vi "Start stream.vi"(10 "Channels to stream":string[](array[string]), 11 "Connection type":string) -> (0 "error out":errorcluster, 1 "ScansPerRead":i32, 2 "Actual ScanRate":dbl format="%.3f", 3 "Handle out":i32, 4 "Number of channels":i32)   [LabVIEW 2018]
panel:
  out "Stream channels":i32[](array[numeric])
  # "This sub VI opens a stream in Labjack. All the settings for the stream are also set here."
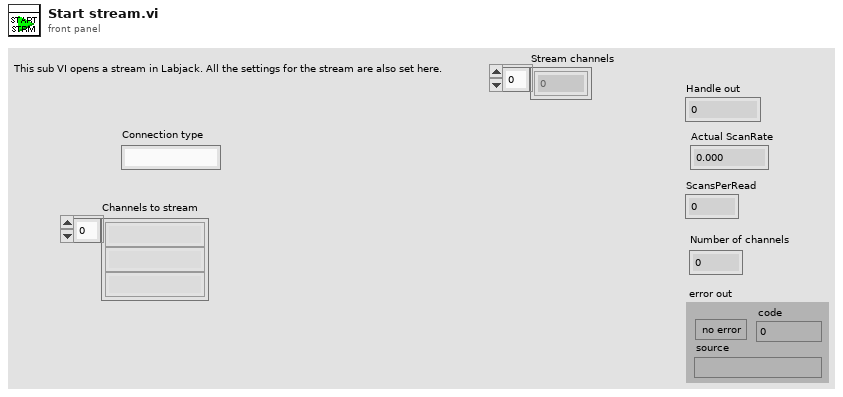
[diagram p1: front panel]
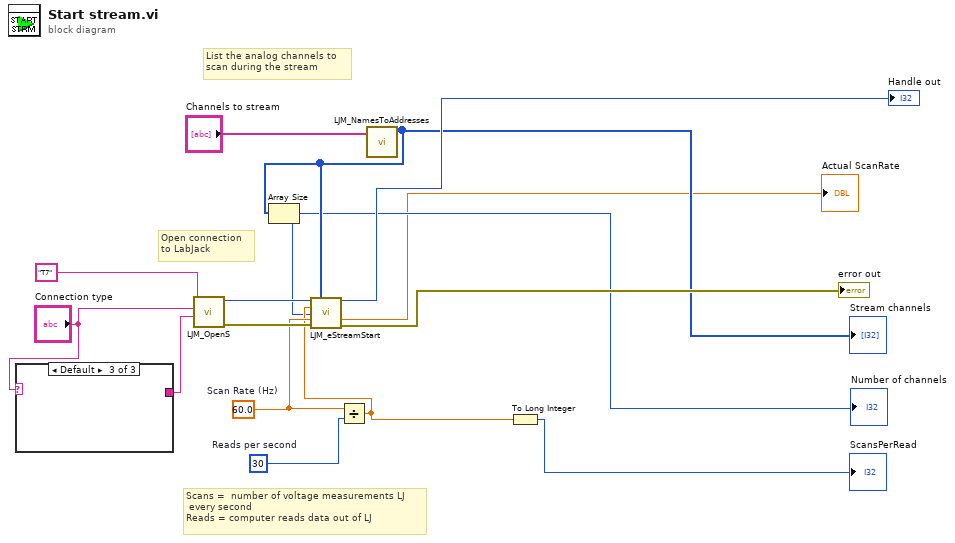
[diagram p0: block diagram]
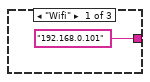
[diagram p2: hidden frame]
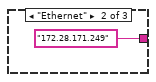
[diagram p3: hidden frame]
diagram:
  w9 = 30  # Reads per second
  w10 = 60.0  # Scan Rate (Hz)
  # "Open connection\nto LabJack"
  # "List the analog channels to \nscan during the stream"
  # "Scans =  number of voltage measurements LJ\n every second\nReads = computer reads data out of LJ"
  n1 = case shown="Default" "Connection type" {
    tunnel: ["192.168.0.101" "172.28.171.249" _] -> w13
    frame "Wifi" {
    }
    frame "Ethernet" {
    }
    frame Default {
    }
  }
  n2 = call "LJM_OpenS.vi"("Identifier"=w13, "ConnectionType"="Connection type", "DeviceType"="T7") -> ("error out"=w11:errorcluster, "Handle"=w12:i32)  [unwired: 7 in]
  n3 = Divide(x=w10, y=w9) -> (x/y=w5:dbl)
  n4 = call "LJM_NamesToAddresses.vi"("aNames"="Channels to stream") -> ("aAddresses"=w6:i32[])  [unwired: 8 in, 2 out]
  "Stream channels" <- w6
  n5 = Array Size(array=w6) -> (size(s)=w3:i32)
  "Number of channels" <- w3
  n6 = call "LJM_eStreamStart.vi"("Handle In"=w12, "aScanList"=w6, "ScansPerRead"=w5, "NumAddresses (Auto-Detect)"=w3, "ScanRate"=w10, "error in"=w11) -> ("Handle Out"=→"Handle out":i32, "Actual ScanRate"=→"Actual ScanRate":dbl, "error out"=→"error out":errorcluster)  [unwired: 4 in, 3 out]
  n7 = To Long Integer(number=w5) -> (32bit integer=→"ScansPerRead":i32)
